vi "Get Keys.vi"(8 "error in (no error)":errorcluster, 10 "section":string, 11 "Configuration Reference In":refnum<data-value>) -> (0 "error out":errorcluster, 1 "key names":string[](array[string]), 2 "section exists?":bool, 3 "Configuration Reference Out":refnum<data-value>)   [LabVIEW 2012, in "configlib.lvlib"]
uses:
  configlib.lvlib
  Configuration File Definition.ctl
  File Options.ctl
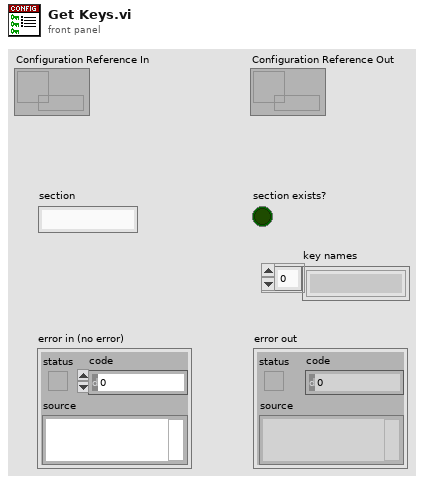
[diagram p1: front panel]
types:
  T1 = typedef "configlib.lvlib/Configuration File Definition.ctl" = cluster{"dirty":bool, "path":path, "Fileopts":T2, "Section Lookup":variant, "Key Lookup":variant, "Raw File":string[]}
  T2 = typedef "configlib.lvlib/File Options.ctl" = cluster{"Name/Value delimiter (\"=\")":string, "Comment delimiter (\";\")":string}
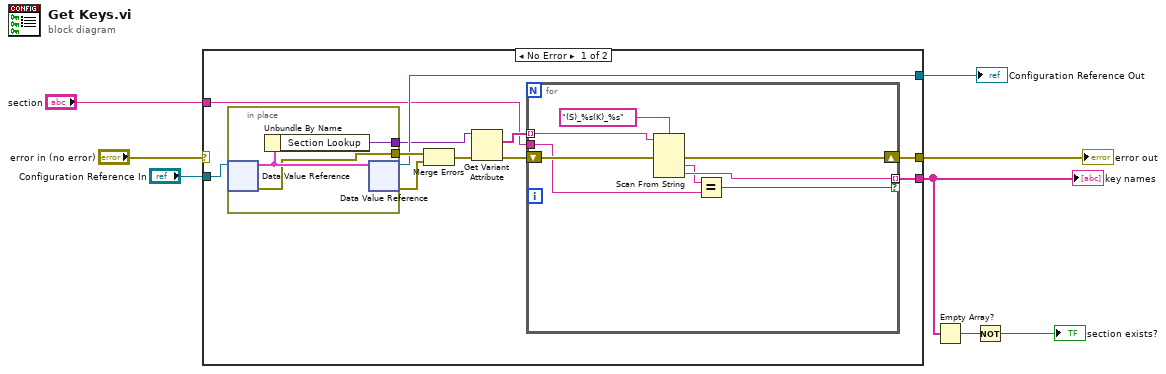
[diagram p0: block diagram]
diagram:
  n1 = case shown="No Error" "error in (no error)" {
    selector: "error in (no error)" -> [_ w32]
    tunnel: [w11 w32] -> w7
    tunnel: "section" -> [w10 _]
    tunnel: "Configuration Reference In" -> [w19 w31]
    tunnel: [w16 w31] -> w4
    tunnel: [w9 _] -> w1
    frame No Error {
      n2 = in-place {
        in-place-border: [w29] -> w14
        in-place-border: [w28] -> w18
        n3 = in-place-dvr #1(w19) -> (w30:T1, w28:errorcluster)
        n4 = Unbundle By Name(w30) -> ("Section Lookup"=w29:variant)
        n5 = in-place-dvr #1(w30) -> (w16:refnum<data-value>, w17:errorcluster)
      }
      n6 = Merge Errors(w18, w17) -> (w15:errorcluster)
      n7 = Get Variant Attribute(Variant=w14, error in=w15) -> (names=w13:string[], error out=w12:errorcluster)  [unwired: 2 in, 2 out]
      n8 = for {
        tunnel: w13 -> [w25] mode=indexing
        shift-right: [w26] -> w11
        shift-left: w12 -> [w27]
        tunnel: [w23] -> w9 mode=indexing if=w20
        tunnel: w10 -> [w22]
        n9 = Scan From String(format string="(S)_%s(K)_%s", input string=w25, error in=w27) -> (error out=w26:errorcluster, output 1=w21:string, output 2=w23:string)  [unwired: 3 in, 2 out]
        n10 = Equal?(x=w21, y=w22) -> (x = y?=w20:bool)
      }
    }
    frame Error {
    }
  }
  "Configuration Reference Out" <- w4
  "error out" <- w7
  "key names" <- w1
  n11 = Empty Array?(array=w1) -> (empty?=w3:bool)
  n12 = Not(x=w3) -> (.not. x?=→"section exists?":bool)
